vi "String - Check Hold Parameters.vi"(9 "Master Data Hold Time (HH:MM)":string, 10 "Master Data Hold Temperature":string, 11 "2D Array in":string[][](array[string])) -> (1 "index of Matched Hold Temperature":i32, 2 "Found":bool, 3 "Message":string)   [LabVIEW 2013]
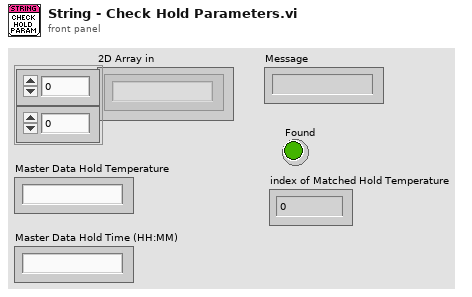
[diagram p1: front panel]
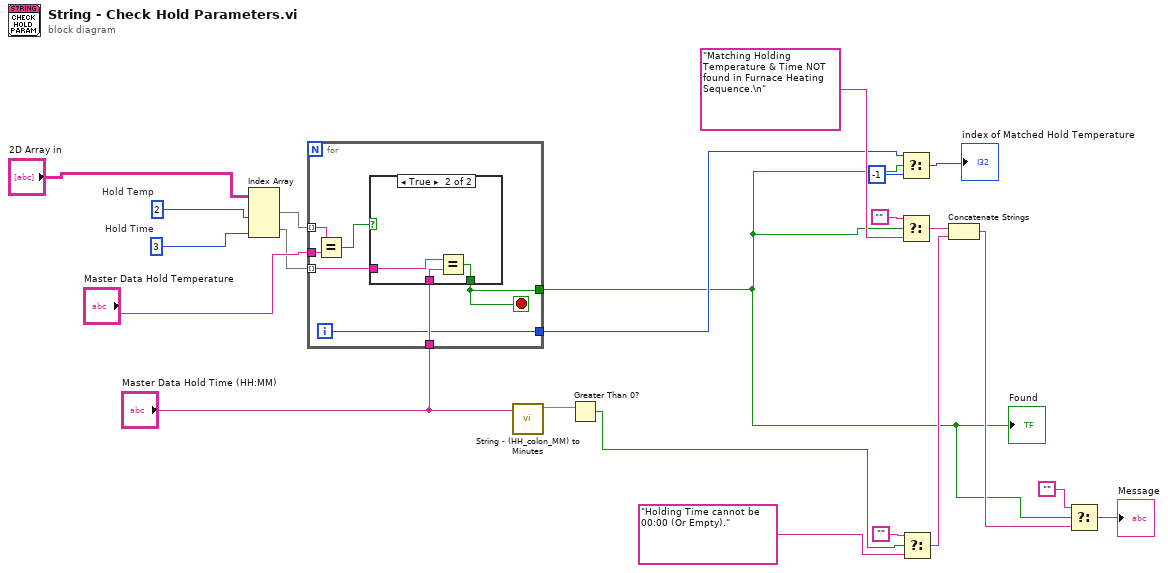
[diagram p0: block diagram]
diagram:
  w8 = 3  # Hold Time
  w16 = 2  # Hold Temp
  n1 = Index Array(array="2D Array in", index (col) #1=w16, index (col) #2=w8) -> (element #1=w9:string[], element #2=w6:string[])  [unwired: 2 in]
  n2 = for {
    tunnel: w9 -> [w29] mode=indexing
    tunnel: "Master Data Hold Temperature" -> [w28]
    tunnel: w6 -> [w26] mode=indexing
    tunnel: "Master Data Hold Time (HH:MM)" -> [w25]
    tunnel: [w24] -> w1
    tunnel: [w23] -> w4
    i -> [w23]
    stop <- w24 stop-if-true
    n3 = Equal?(x=w29, y=w28) -> (x = y?=w27:bool)
    n4 = case shown="True" w27 {
      tunnel: w26 -> [_ w32]
      tunnel: w25 -> [_ w31]
      tunnel: [_ w30] -> w24
      frame False {
      }
      frame True {
        n5 = Equal?(x=w32, y=w31) -> (x = y?=w30:bool)
      }
    }
  }
  "Found" <- w1
  n6 = call "String - (HH_colon_MM) to Minutes.vi"("Hold Time (HH:MM)"="Master Data Hold Time (HH:MM)") -> ("minutes"=w12:dbl)  [unwired: 10 in]
  n7 = Greater Than 0?(x=w12) -> (x > 0?=w11:bool)
  n8 = Select(t=w4, s=w1, f=-1) -> (s? t:f=→"index of Matched Hold Temperature":i32)
  n9 = Select(t="", s=w1, f="Matching Holding Temperature & Time NOT found in Furnace Heating Sequence.\n" ("string")) -> (s? t:f=w20:string)
  n10 = Select(t="", s=w11, f="Holding Time cannot be 00:00 (Or Empty)." ("string")) -> (s? t:f=w17:string)
  n11 = Concatenate Strings(w20, w17) -> (w14:string)
  n12 = Select(t="", s=w1, f=w14) -> (s? t:f=→"Message":string)
